vi "Exact Match Pattern.vi"(10 "Pattern":string) -> (2 "Exact Match Pattern":string)   [LabVIEW 2020, in "CDM-Config.lvlib"]
uses:
  CDM-Config.lvlib
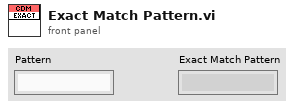
[diagram p1: front panel]
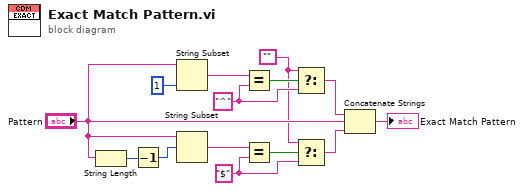
[diagram p0: block diagram]
diagram:
  w1 = ""
  w6 = "$" ("y")
  w9 = "^" ("y")
  n1 = String Length(string="Pattern") -> (length=w13:i32)
  n2 = Decrement(x=w13) -> (x-1=w12:i32)
  n3 = String Subset(string="Pattern", length (rest)=1 ("length (rest)")) -> (substring=w11:string)  [unwired: 1 in]
  n4 = String Subset(string="Pattern", offset (0)=w12) -> (substring=w4:string)  [unwired: 1 in]
  n5 = Equal?(x=w11, y=w9) -> (x = y?=w10:bool)
  n6 = Equal?(x=w4, y=w6) -> (x = y?=w5:bool)
  n7 = Select(t=w1, s=w10, f=w9) -> (s? t:f=w7:string)
  n8 = Select(t=w1, s=w5, f=w6) -> (s? t:f=w3:string)
  n9 = Concatenate Strings(w7, "Pattern", w3) -> (→"Exact Match Pattern":string)
